vi "CollatzConjecture.vi"() -> ()   [LabVIEW 2019]
panel:
  out "Array":dbl[](array[numeric])
  in  "Numeric":i32 min=0 max=1000 step=1
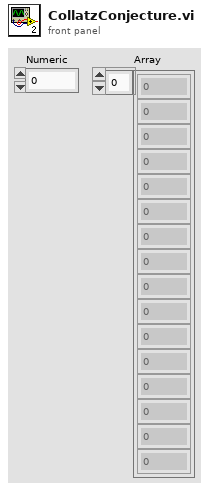
[diagram p1: front panel]
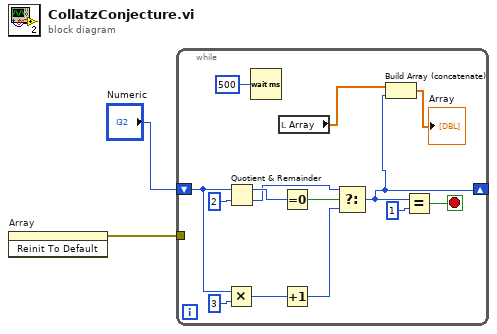
[diagram p0: block diagram]
diagram:
  n1 = invoke on="Array" class="Arr (strict)" method="Reinit To Default"() -> (error out=w1:errorcluster)  [unwired: 3 in, 2 out]
  n2 = while {
    shift-right: [w4] -> _
    shift-left: "Numeric" -> [w13]
    tunnel: w1 -> [_]
    stop <- w8 stop-if-true
    n3 = Multiply(x=w13, y=3) -> (x*y=w11:i32)
    n4 = Quotient & Remainder(x=w13, y=2) -> (x-y*floor(x/y)=w7:i32, floor(x/y)=w6:i32)
    n5 = Wait (ms)(milliseconds to wait=u32 500) -> ()  [unwired: 1 out]
    n6 = local read "Array"() -> (w5:dbl[])
    n7 = Equal To 0?(x=w7) -> (x = 0?=w14:bool)
    n8 = Increment(x=w11) -> (x+1=w10:i32)
    n9 = Select(t=w6, s=w14, f=w10) -> (s? t:f=w4:i32)
    n10 = Build Array (concatenate)(w5, w4) -> (→"Array":dbl[])
    n11 = Equal?(x=w4, y=1) -> (x = y?=w8:bool)
  }
